vi "onAssertionSlippage.vi"(7 "TraceabilityMatrix in":refnum<class "TraceabilityMatrix.lvclass">, 11 "Leaf.Assertion":refnum<class "Leaf.Assertion.lvclass">) -> (0 "error out":errorcluster, 3 "Leaf.Assertion":refnum<class "Leaf.Assertion.lvclass">)   [LabVIEW 2021, in "Bananas.lvlib" / "TraceabilityMatrix.lvclass"]
uses:
  TraceabilityMatrix.lvclass
  Leaf.Assertion/Leaf.Assertion.lvclass
  C:/Repositories/LVOS/Bananas/lv-src/Bananas/Leaf/Leaf.lvclass
  TraceabilityMatrix.lvclass/TraceabilityMatrix.ctl
  Leaf/Leaf.lvclass
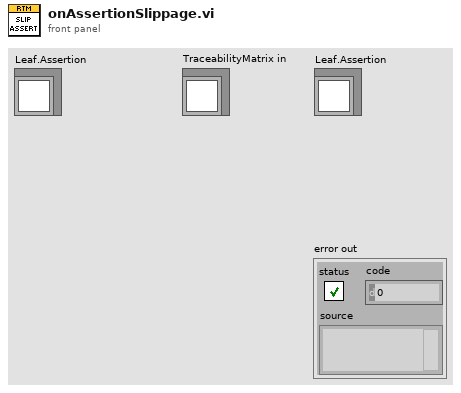
[diagram p1: front panel]
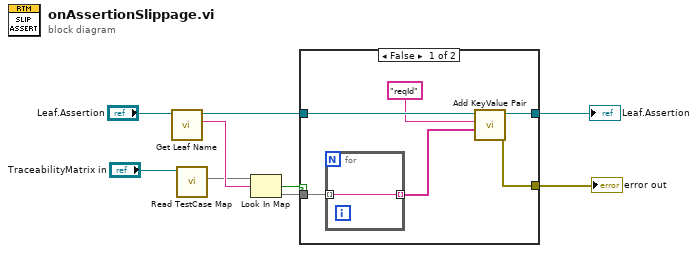
[diagram p0: block diagram]
diagram:
  n1 = call "Get Leaf Name.vi"("Leaf in"="Leaf.Assertion") -> ("Name"=w4:string, "Leaf out"=w3:refnum<class "Leaf.Assertion.lvclass">)  [unwired: 8 in, 1 out]
  n2 = call "Read TestCase Map.vi"("TraceabilityMatrix in"="TraceabilityMatrix in") -> ("TestCaseMap"=w1:map{string, set{string}})  [unwired: 9 in, 1 out]
  n3 = Look In Map(map=w1, key=w4) -> (key not found?=w9:bool, value=w7:set{string})  [unwired: 1 in]
  n4 = case shown="False" w9 {
    tunnel: [w13 w17] -> w8
    tunnel: w3 -> [w15 w17]
    tunnel: w7 -> [w11 _]
    tunnel: [w12 _] -> w6
    frame False {
      n5 = for {
        tunnel: w11 -> [w16] mode=indexing
        tunnel: [w16] -> w10 mode=indexing
      }
      n6 = call "Add KeyValue Pair.vi"("value"=w10, "key"="reqId", "Leaf in"=w15) -> ("error out"=w12:errorcluster, "Leaf out"=w13:refnum<class "Leaf.Assertion.lvclass">)  [unwired: 7 in]
    }
    frame True {
    }
  }
  "error out" <- w6
  "Leaf.Assertion" <- w8
